vi "Get All AttributeName and Value.vi"(8 "error in (no error)":errorcluster, 10 "AttributeNames(\"\")":string[](array[string]), 11 "Part in":refnum<class "Part.lvclass">) -> (0 "error out":errorcluster, 2 "AttributeValues":variant[](array[variant]), 3 "Part out":refnum<class "Part.lvclass">)   [LabVIEW 2015, in "Part.lvclass"]
uses:
  Part.lvclass
  Part.lvclass/Part.ctl
  <vilib>/Utility/error.llb/Error Cluster From Error Code.vi
  <vilib>/ErrorRing/Error Ring.xnode
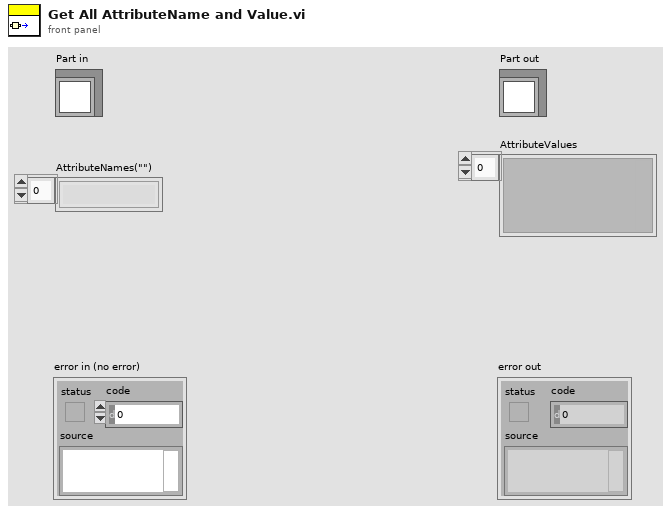
[diagram p1: front panel]
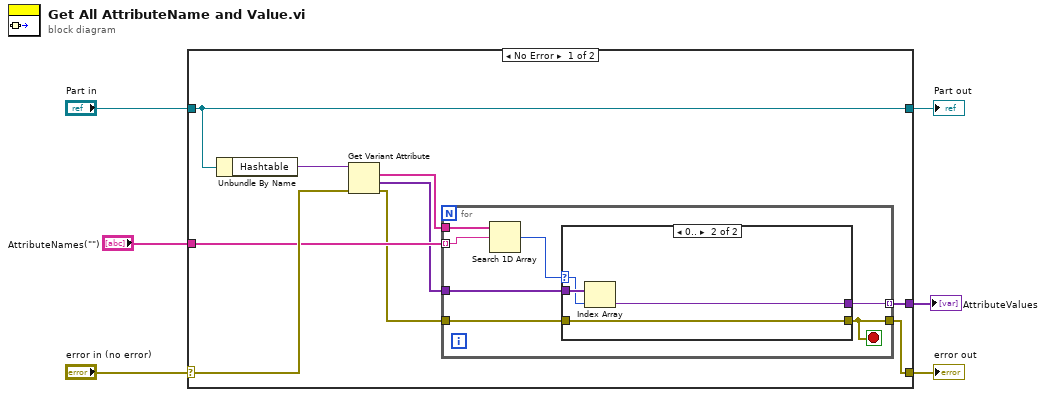
[diagram p0: block diagram]
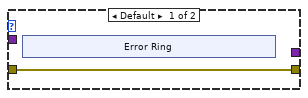
[diagram p2: hidden frame]
diagram:
  n1 = case shown="No Error" "error in (no error)" {
    selector: "error in (no error)" -> [w13 w34]
    tunnel: [w8 w34] -> w5
    tunnel: [w15 w33] -> w3
    tunnel: "Part in" -> [w15 w33]
    tunnel: "AttributeNames(\"\")" -> [w12 _]
    tunnel: [w7 _] -> w1
    frame No Error {
      n2 = Unbundle By Name(w15) -> ("Hashtable"=w14:variant)
      n3 = Get Variant Attribute(Variant=w14, error in=w13) -> (names=w11:string[], values=w10:variant[], error out=w9:errorcluster)  [unwired: 2 in, 1 out]
      n4 = for {
        tunnel: w12 -> [w21] mode=indexing
        tunnel: w11 -> [w22]
        tunnel: w10 -> [w20]
        tunnel: [w19] -> w7 mode=indexing
        tunnel: w9 -> [w17]
        tunnel: [w16] -> w8
        stop <- w16 stop-if-true
        n5 = Search 1D Array(1D array=w22, element=w21) -> (index of element=w18:i32)  [unwired: 1 in]
        n6 = case shown="0.." w18 {
          selector: w18 -> [_ w30]
          tunnel: w20 -> [_ w32]
          tunnel: [_ w31] -> w19
          tunnel: w17 -> [w23 w29]
          tunnel: [w23 w29] -> w16
          frame Default {
            n7 = xnode "Error Ring"() -> ()  [unwired: 1 out]
          }
          frame 0.. {
            n8 = Index Array(array=w32, index=w30) -> (element=w31:variant)
          }
        }
      }
    }
    frame Error {
    }
  }
  "error out" <- w5
  "Part out" <- w3
  "AttributeValues" <- w1
